vi "Jasco_UVvis.vi"() -> ()   [LabVIEW 2018]
uses:
  <vilib>/Instr/_visa.llb/VISA Configure Serial Port (Instr).vi
panel:
  in  "?":T1(tab)
  out "?":ext(graph)
  in  "SW read":bool
  out "Absorbance (ABU)":dbl
  in  "Sample rate (ms)":dbl=500.0
  in  "Wavelength (nm)":i32=350
  in  "Single wavelength absorbtion file path":path
  out "?":T2(graph)
  in  "Measure background spectra":bool
  in  "read spectrum":bool
  in  "Single wavelength absorbtion file path 2":path
  in  "stop 3":bool
  in  "stop 2":bool
  in  "flow control (0:none)":u16(ring)=1 items=["None", "XON/XOFF", "RTS/CTS", "XON/XOFF & RTS/CTS", "DTR/DSR", "XON/XOFF & DTR/DSR"]
  in  "stop bits (10: 1 bit)":u16(ring)=20 items=["1.0"=10, "1.5"=15, "2.0"=20]
  in  "parity (0:none)":enum16{"None", "Odd", "Even", "Mark", "Space"}(ring)
  in  "data bits (8)":u16=8 min=5 max=8 step=1
  in  "baud rate (9600)":u32=4800
  in  "VISA resource name":refnum<visa-resource-name>="COM4"
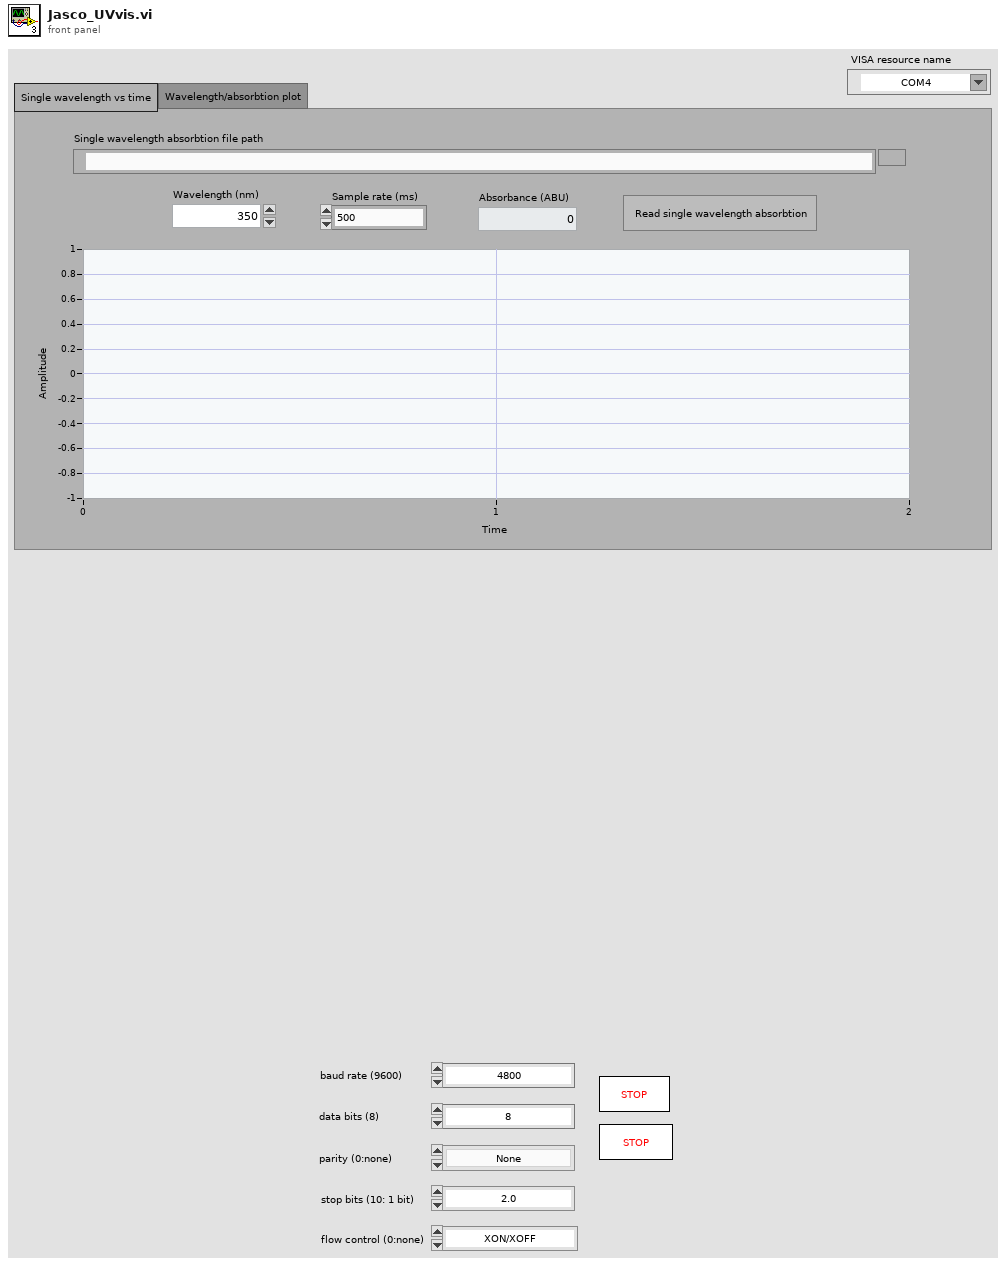
[diagram p1: front panel]
types:
  T1 = enum32{"Single wavelength vs time", "Wavelength/absorbtion plot"}
  T2 = cluster{"array type (2D Dbl)":dbl[], "array type (2D Dbl)":dbl[]}
  T3 = enum16{"open", "replace", "create", "open or create", "replace or create", "replace or create with confirmation"}
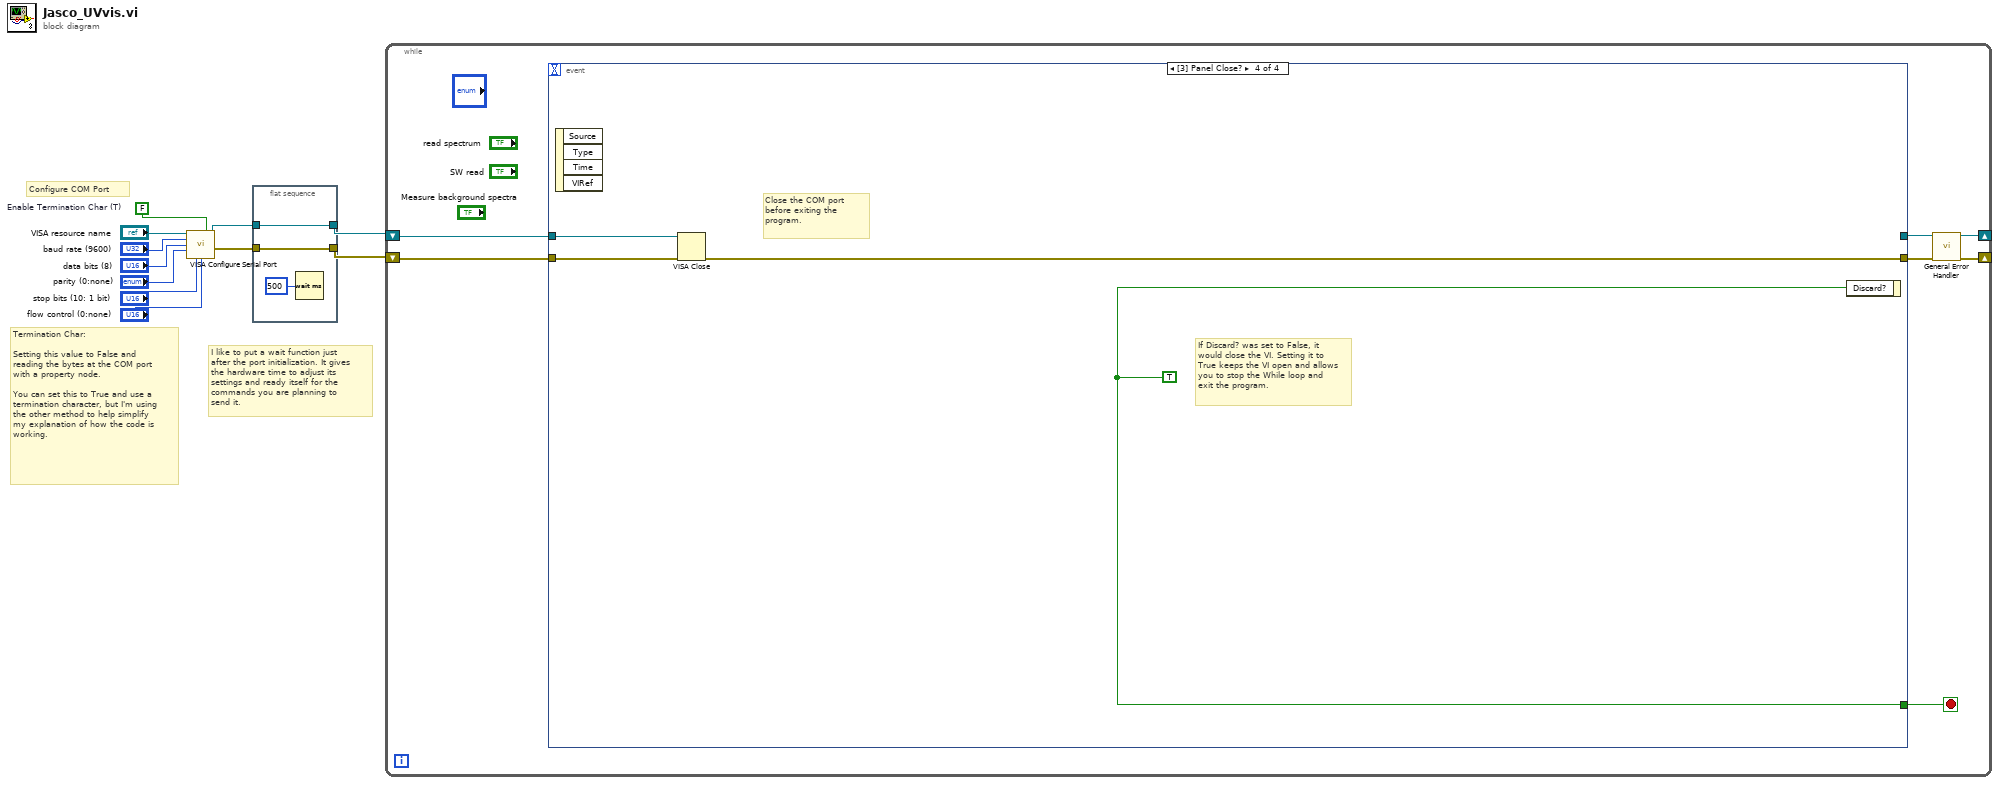
[diagram p0: block diagram]
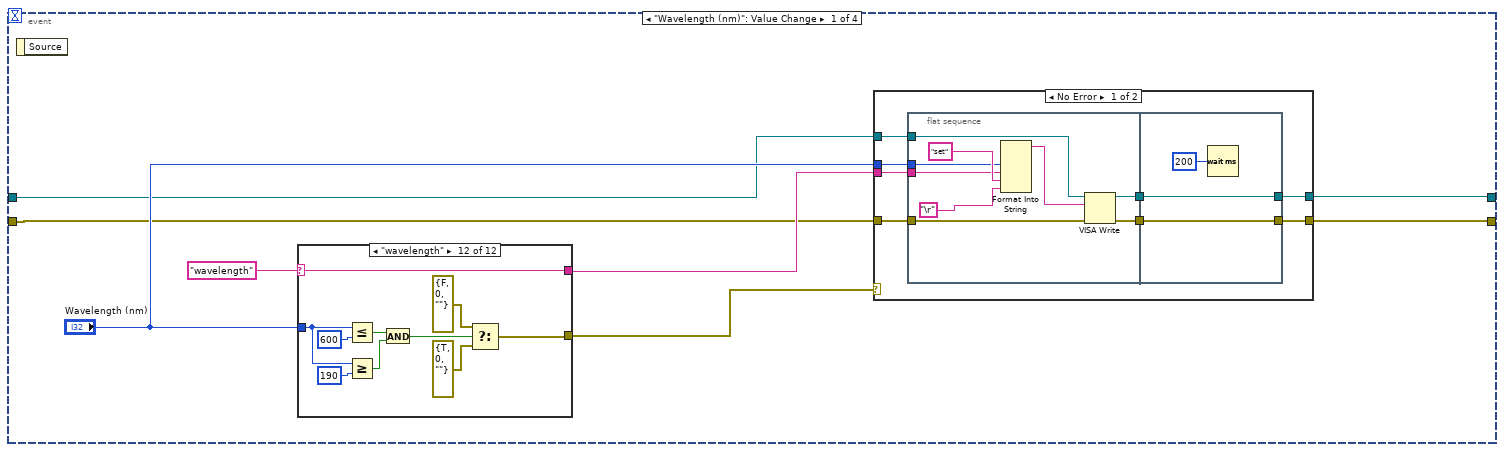
[diagram p2: hidden frame]
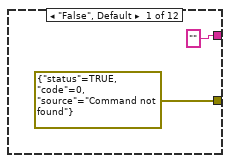
[diagram p4: hidden frame]
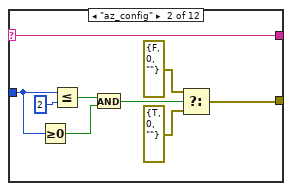
[diagram p5: hidden frame]
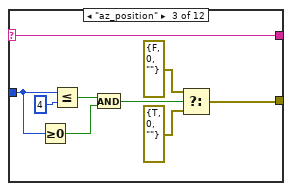
[diagram p6: hidden frame]
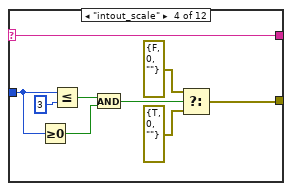
[diagram p7: hidden frame]
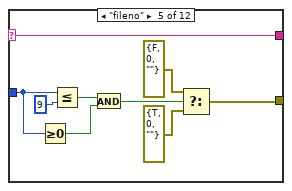
[diagram p8: hidden frame]
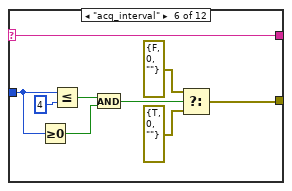
[diagram p9: hidden frame]
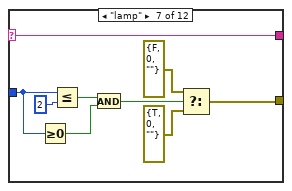
[diagram p10: hidden frame]
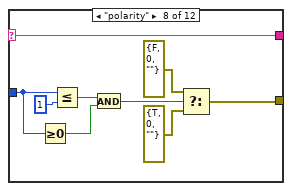
[diagram p11: hidden frame]
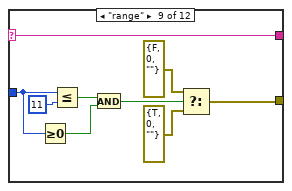
[diagram p12: hidden frame]
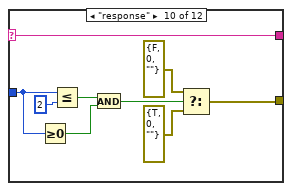
[diagram p13: hidden frame]
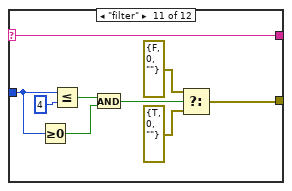
[diagram p14: hidden frame]
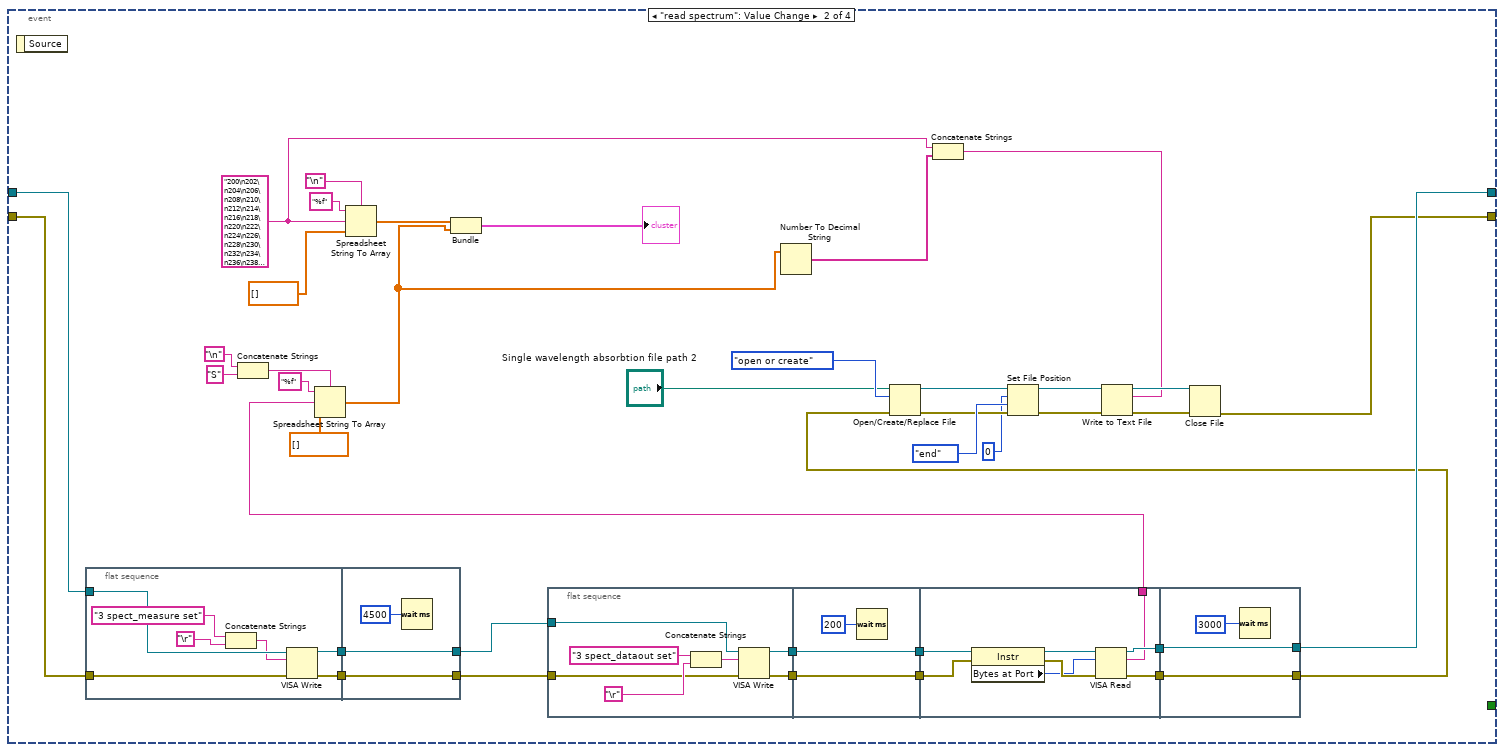
[diagram p15: hidden frame]
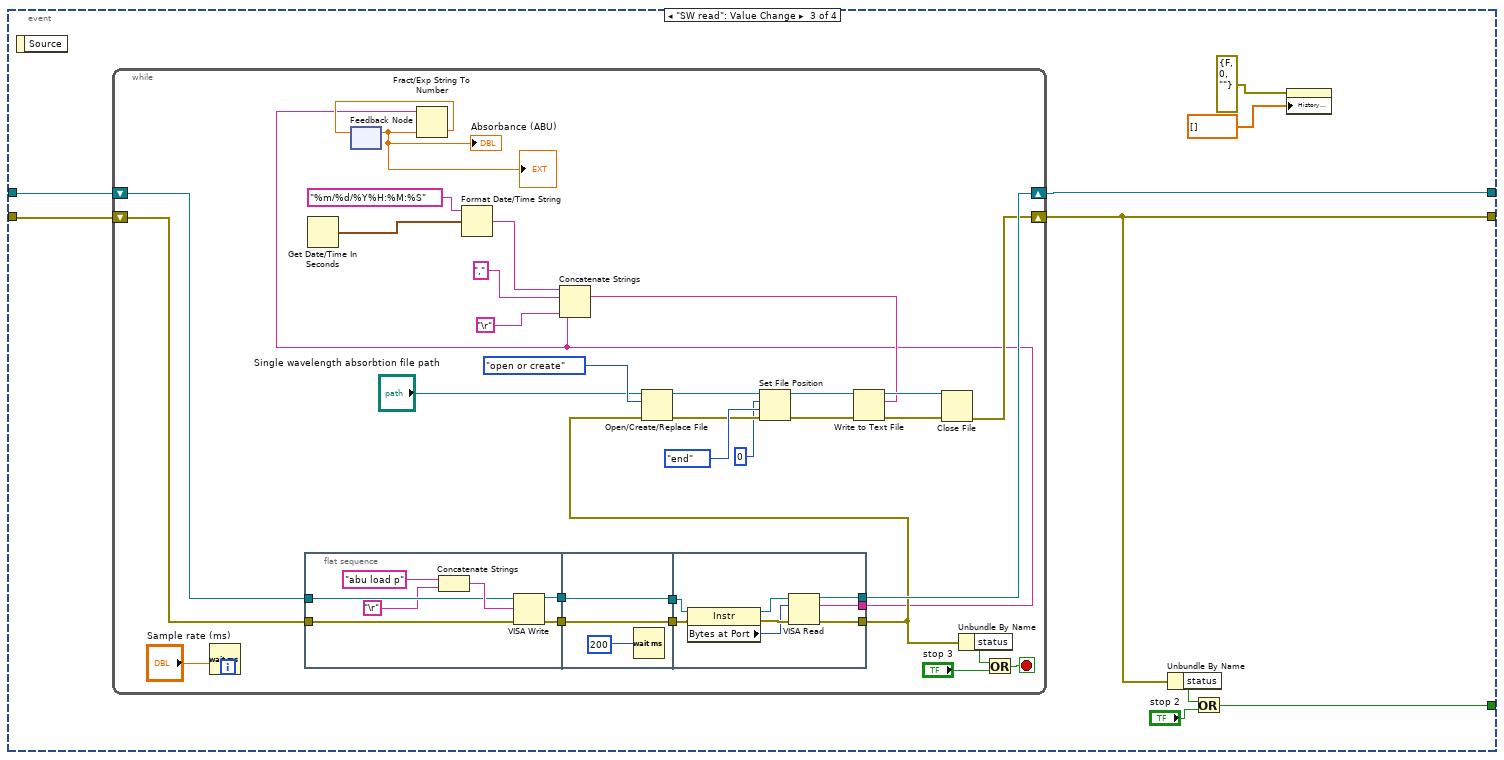
[diagram p16: hidden frame]
diagram:
  w5 = FALSE  # Enable Termination Char (T)
  # "Termination Char:\n\nSetting this value to False and reading the bytes at the COM port with a property node.\n\nYou can set this to True and use a termination character, but I'm using the other method to help simplify my explanation of how the code is working."
  # "I like to put a wait function just after the port initialization. It gives the hardware time to adjust its settings and ready itself for the commands you are planning to send it."
  # "Configure COM Port"
  n1 = call-poly "VISA Configure Serial Port"("VISA resource name"="VISA resource name", "Enable Termination\nChar (T)"=w5, "baud rate (9600)"="baud rate (9600)", "data bits (8)"="data bits (8)", "parity (0:none)"="parity (0:none)", "stop bits (10: 1 bit)"="stop bits (10: 1 bit)", "flow control (0:none)"="flow control (0:none)") -> ("VISA resource name out"=w3:refnum<visa-resource-name>, "error out"=w4:errorcluster)  [unwired: 7 in]
  n2 = flat-sequence {
    tunnel: [w13] -> w1
    tunnel: w4 -> [w13]
    tunnel: [w12] -> w2
    tunnel: w3 -> [w12]
    frame #0 {
      n3 = Wait (ms)(milliseconds to wait=u32 500) -> ()  [unwired: 1 out]
    }
  }
  n4 = while {
    shift-right: [w18] -> _
    shift-left: w2 -> [w20]
    shift-right: [w16] -> _
    shift-left: w1 -> [w19]
    stop <- w15 stop-if-true
    n5 = event shown="[3] Panel Close?" {
      selector: _ -> [_ _ _ _]
      dyn-events: _ -> [_ _ _ _]
      timeout: _ -> [_ _ _ _]
      tunnel: w20 -> [w24 w186 w231 w286]
      tunnel: w19 -> [w23 w184 w230 w285]
      tunnel: [w22 w157 w226 w284] -> w17
      tunnel: [w21 w182 w232 _] -> w18
      tunnel: [_ _ w227 w283] -> w15
      event "Wavelength (nm)": Value Change {
        n6 = event-data() -> ()  [unwired: 1 in, 1 out]
        n7 = case shown="\"wavelength\"" "wavelength" {
          selector: "wavelength" -> [_ w61 w70 w79 w88 w97 w106 w115 w124 w133 w142 w152]
          tunnel: ["" w61 w70 w79 w88 w97 w106 w115 w124 w133 w142 w152] -> w27
          tunnel: "Wavelength (nm)" -> [_ w60 w69 w78 w87 w96 w105 w114 w123 w132 w141 w144]
          tunnel: [errorcluster {"status"=TRUE, "code"=0, "source"="Command not found"} ("error in (no error)") w53 w62 w71 w80 w89 w98 w107 w116 w125 w134 w145] -> w28
          frame "False", Default {
          }
          frame "az_config" {
            n8 = Greater Or Equal To 0?(x=w60) -> (x >= 0?=w57:bool)
            n9 = Less Or Equal?(x=w60, y=2) -> (x <= y?=w58:bool)
            n10 = And(x=w58, y=w57) -> (x .and. y?=w56:bool)
            n11 = Select(t=errorcluster {"status"=FALSE, "code"=0, "source"=""} ("error in (no error)"), s=w56, f=errorcluster {"status"=TRUE, "code"=0, "source"=""} ("error in (no error)")) -> (s? t:f=w53:errorcluster)
          }
          frame "az_position" {
            n12 = Greater Or Equal To 0?(x=w69) -> (x >= 0?=w66:bool)
            n13 = Less Or Equal?(x=w69, y=4) -> (x <= y?=w67:bool)
            n14 = And(x=w67, y=w66) -> (x .and. y?=w65:bool)
            n15 = Select(t=errorcluster {"status"=FALSE, "code"=0, "source"=""} ("error in (no error)"), s=w65, f=errorcluster {"status"=TRUE, "code"=0, "source"=""} ("error in (no error)")) -> (s? t:f=w62:errorcluster)
          }
          frame "intout_scale" {
            n16 = Greater Or Equal To 0?(x=w78) -> (x >= 0?=w75:bool)
            n17 = Less Or Equal?(x=w78, y=3) -> (x <= y?=w76:bool)
            n18 = And(x=w76, y=w75) -> (x .and. y?=w74:bool)
            n19 = Select(t=errorcluster {"status"=FALSE, "code"=0, "source"=""} ("error in (no error)"), s=w74, f=errorcluster {"status"=TRUE, "code"=0, "source"=""} ("error in (no error)")) -> (s? t:f=w71:errorcluster)
          }
          frame "fileno" {
            n20 = Greater Or Equal To 0?(x=w87) -> (x >= 0?=w84:bool)
            n21 = Less Or Equal?(x=w87, y=9) -> (x <= y?=w85:bool)
            n22 = And(x=w85, y=w84) -> (x .and. y?=w83:bool)
            n23 = Select(t=errorcluster {"status"=FALSE, "code"=0, "source"=""} ("error in (no error)"), s=w83, f=errorcluster {"status"=TRUE, "code"=0, "source"=""} ("error in (no error)")) -> (s? t:f=w80:errorcluster)
          }
          frame "acq_interval" {
            n24 = Greater Or Equal To 0?(x=w96) -> (x >= 0?=w93:bool)
            n25 = Less Or Equal?(x=w96, y=4) -> (x <= y?=w94:bool)
            n26 = And(x=w94, y=w93) -> (x .and. y?=w92:bool)
            n27 = Select(t=errorcluster {"status"=FALSE, "code"=0, "source"=""} ("error in (no error)"), s=w92, f=errorcluster {"status"=TRUE, "code"=0, "source"=""} ("error in (no error)")) -> (s? t:f=w89:errorcluster)
          }
          frame "lamp" {
            n28 = Greater Or Equal To 0?(x=w105) -> (x >= 0?=w102:bool)
            n29 = Less Or Equal?(x=w105, y=2) -> (x <= y?=w103:bool)
            n30 = And(x=w103, y=w102) -> (x .and. y?=w101:bool)
            n31 = Select(t=errorcluster {"status"=FALSE, "code"=0, "source"=""} ("error in (no error)"), s=w101, f=errorcluster {"status"=TRUE, "code"=0, "source"=""} ("error in (no error)")) -> (s? t:f=w98:errorcluster)
          }
          frame "polarity" {
            n32 = Greater Or Equal To 0?(x=w114) -> (x >= 0?=w111:bool)
            n33 = Less Or Equal?(x=w114, y=1) -> (x <= y?=w112:bool)
            n34 = And(x=w112, y=w111) -> (x .and. y?=w110:bool)
            n35 = Select(t=errorcluster {"status"=FALSE, "code"=0, "source"=""} ("error in (no error)"), s=w110, f=errorcluster {"status"=TRUE, "code"=0, "source"=""} ("error in (no error)")) -> (s? t:f=w107:errorcluster)
          }
          frame "range" {
            n36 = Greater Or Equal To 0?(x=w123) -> (x >= 0?=w120:bool)
            n37 = Less Or Equal?(x=w123, y=11) -> (x <= y?=w121:bool)
            n38 = And(x=w121, y=w120) -> (x .and. y?=w119:bool)
            n39 = Select(t=errorcluster {"status"=FALSE, "code"=0, "source"=""} ("error in (no error)"), s=w119, f=errorcluster {"status"=TRUE, "code"=0, "source"=""} ("error in (no error)")) -> (s? t:f=w116:errorcluster)
          }
          frame "response" {
            n40 = Greater Or Equal To 0?(x=w132) -> (x >= 0?=w129:bool)
            n41 = Less Or Equal?(x=w132, y=2) -> (x <= y?=w130:bool)
            n42 = And(x=w130, y=w129) -> (x .and. y?=w128:bool)
            n43 = Select(t=errorcluster {"status"=FALSE, "code"=0, "source"=""} ("error in (no error)"), s=w128, f=errorcluster {"status"=TRUE, "code"=0, "source"=""} ("error in (no error)")) -> (s? t:f=w125:errorcluster)
          }
          frame "filter" {
            n44 = Greater Or Equal To 0?(x=w141) -> (x >= 0?=w138:bool)
            n45 = Less Or Equal?(x=w141, y=4) -> (x <= y?=w139:bool)
            n46 = And(x=w139, y=w138) -> (x .and. y?=w137:bool)
            n47 = Select(t=errorcluster {"status"=FALSE, "code"=0, "source"=""} ("error in (no error)"), s=w137, f=errorcluster {"status"=TRUE, "code"=0, "source"=""} ("error in (no error)")) -> (s? t:f=w134:errorcluster)
          }
          frame "wavelength" {
            n48 = Less Or Equal?(x=w144, y=600) -> (x <= y?=w150:bool)
            n49 = Greater Or Equal?(x=w144, y=190) -> (x >= y?=w149:bool)
            n50 = And(x=w150, y=w149) -> (x .and. y?=w148:bool)
            n51 = Select(t=errorcluster {"status"=FALSE, "code"=0, "source"=""} ("error in (no error)"), s=w148, f=errorcluster {"status"=TRUE, "code"=0, "source"=""} ("error in (no error)")) -> (s? t:f=w145:errorcluster)
          }
        }
        n52 = case shown="No Error" w28 {
          tunnel: w24 -> [w34 w49]
          tunnel: [w33 w49] -> w21
          tunnel: [w32 w50] -> w22
          tunnel: w23 -> [w31 w50]
          tunnel: w27 -> [w30 _]
          tunnel: "Wavelength (nm)" -> [w29 _]
          frame No Error {
            n53 = flat-sequence {
              tunnel: w30 -> [w39]
              tunnel: w31 -> [w45]
              tunnel: w34 -> [w44]
              tunnel: [w43] -> w36
              tunnel: [w42] -> w35
              tunnel: w29 -> [w38]
              tunnel: [w47] -> w32
              tunnel: w36 -> [w47]
              tunnel: [w46] -> w33
              tunnel: w35 -> [w46]
              frame #0 {
                n54 = Format Into String(w38, w39, "set" ("string"), "\r") -> (resulting string=w40:string)  [unwired: 3 in, 1 out]
                n55 = VISA Write(VISA resource name=w44, write buffer=w40, error in (no error)=w45) -> (VISA resource name out=w42:refnum<visa-resource-name>, error out=w43:errorcluster)  [unwired: 1 out]
              }
              frame #1 {
                n56 = Wait (ms)(milliseconds to wait=u32 200) -> ()  [unwired: 1 out]
              }
            }
          }
          frame Error {
          }
        }
      }
      event "read spectrum": Value Change {
        w156 = "200\n202\n204\n206\n208\n210\n212\n214\n216\n218\n220\n222\n224\n226\n228\n230\n232\n234\n236\n238\n240\n242\n244\n246\n248\n250\n252\n254\n256\n258\n260\n262\n264\n266\n268\n270\n272\n274\n276\n278\n280\n282\n284\n286\n288\n290\n292\n294\n296\n298\n300\n302\n304\n306\n308\n310\n312\n314\n316\n318\n320\n322\n324\n326\n328\n330\n332\n334\n336\n338\n340\n342\n344\n346\n348\n350\n352\n354\n356\n358\n360\n362\n364\n366\n368\n370\n372\n374\n376\n378\n380\n382\n384\n386\n388\n390\n392\n394\n396\n398\n400\n402\n404\n406\n408\n410\n412\n414\n416\n418\n420\n422\n424\n426\n428\n430\n432\n434\n436\n438\n440\n442\n444\n446\n448\n450\n452\n454\n456\n458\n460\n462\n464\n466\n468\n470\n472\n474\n476\n478\n480\n482\n484\n486\n488\n490\n492\n494\n496\n498\n500\n502\n504\n506\n508\n510\n512\n514\n516\n518\n520\n522\n524\n526\n528\n530\n532\n534\n536\n538\n540\n542\n544\n546\n548\n550\n552\n554\n556\n558\n560\n562\n564\n566\n568\n570\n572\n574\n576\n578\n580\n582\n584\n586\n588\n590\n592\n594\n596\n598\n600\n602\n"
        n57 = event-data() -> ()  [unwired: 1 in, 1 out]
        n58 = flat-sequence {
          tunnel: w184 -> [w199]
          tunnel: w186 -> [w198]
          tunnel: [w197] -> w188
          tunnel: [w196] -> w187
          tunnel: [w201] -> w183
          tunnel: w188 -> [w201]
          tunnel: [w200] -> w185
          tunnel: w187 -> [w200]
          frame #0 {
            n59 = Concatenate Strings("3 spect_measure set" ("string"), "\r") -> (w194:string)
            n60 = VISA Write(VISA resource name=w198, write buffer=w194, error in (no error)=w199) -> (VISA resource name out=w196:refnum<visa-resource-name>, error out=w197:errorcluster)  [unwired: 1 out]
          }
          frame #1 {
            n61 = Wait (ms)(milliseconds to wait=u32 4500) -> ()  [unwired: 1 out]
          }
        }
        n62 = Concatenate Strings("\n", "S") -> (w176:string)
        n63 = Spreadsheet String To Array(delimiter (Tab)=w176, format string="%f", spreadsheet string=w169, array type (2D Dbl)=dbl[] []) -> (array=w155:dbl[])
        n64 = Spreadsheet String To Array(delimiter (Tab)="\n", format string="%f", spreadsheet string=w156, array type (2D Dbl)=dbl[] []) -> (array=w170:dbl[])
        n65 = Bundle("array type (2D Dbl)"=w170, "array type (2D Dbl)"=w155) -> (→"?":T2)  [unwired: 1 in]
        n66 = flat-sequence {
          tunnel: [w207] -> w192
          tunnel: [w206] -> w191
          tunnel: w183 -> [w203]
          tunnel: w185 -> [w208]
          tunnel: w192 -> [w211]
          tunnel: w191 -> [w210]
          tunnel: [w211] -> w190
          tunnel: [w210] -> w189
          tunnel: w190 -> [w220]
          tunnel: w189 -> [w218]
          tunnel: [w216] -> w181
          tunnel: [w214] -> w180
          tunnel: [w213] -> w169
          tunnel: [w222] -> w158
          tunnel: [w223] -> w182
          tunnel: w181 -> [w223]
          tunnel: w180 -> [w222]
          frame #0 {
            n67 = Concatenate Strings("3 spect_dataout set" ("string"), "\r") -> (w209:string)
            n68 = VISA Write(VISA resource name=w208, write buffer=w209, error in (no error)=w203) -> (VISA resource name out=w206:refnum<visa-resource-name>, error out=w207:errorcluster)  [unwired: 1 out]
          }
          frame #1 {
            n69 = Wait (ms)(milliseconds to wait=u32 200) -> ()  [unwired: 1 out]
          }
          frame #2 {
            n70 = property class="Instr"(reference=w218, error in=w220) -> (reference out=w217:refnum<visa-resource-name>, error out=w219:errorcluster, "Bytes at Port"=w215:u32)
            n71 = VISA Read(VISA resource name=w217, byte count=w215, error in (no error)=w219) -> (VISA resource name out=w216:refnum<visa-resource-name>, read buffer=w213:string, error out=w214:errorcluster)  [unwired: 1 out]
          }
          frame #3 {
            n72 = Wait (ms)(milliseconds to wait=u32 3000) -> ()  [unwired: 1 out]
          }
        }
        n73 = Number To Decimal String(number=w155) -> (decimal integer string=w154:string[])  [unwired: 1 in]
        n74 = Open/Create/Replace File(file path (use dialog)="Single wavelength absorbtion file path 2", error in=w158, operation (0:open)=T3."open or create") -> (refnum out=w162:refnum<file>, error out=w161:errorcluster)  [unwired: 3 in, 1 out]
        n75 = Concatenate Strings(w156, w154) -> (w153:string)
        n76 = Set File Position(offset (in bytes) (0)=i64 0, refnum=w162, from (0:start)=enum16{"start", "end", "current"}."end", error in=w161) -> (refnum out=w166:refnum<file>, error out=w167:errorcluster)
        n77 = Write to Text File(file (use dialog)=w166, text=w153, error in=w167) -> (refnum out=w164:refnum<file>, error out=w165:errorcluster)  [unwired: 1 in, 1 out]
        n78 = Close File(refnum=w164, error in=w165) -> (error out=w157:errorcluster)  [unwired: 1 out]
      }
      event "SW read": Value Change {
        n79 = event-data() -> ()  [unwired: 1 in, 1 out]
        n80 = while {
          shift-right: [w260] -> w232
          shift-left: w231 -> [w233]
          shift-right: [w241] -> w226
          shift-left: w230 -> [w238]
          stop <- w257 stop-if-true
          n81 = Wait (ms)(milliseconds to wait="Sample rate (ms)") -> ()  [unwired: 1 out]
          n82 = flat-sequence {
            tunnel: w238 -> [w265]
            tunnel: w233 -> [w270]
            tunnel: [w269] -> w264
            tunnel: [w268] -> w263
            tunnel: w264 -> [w273]
            tunnel: w263 -> [w272]
            tunnel: [w273] -> w262
            tunnel: [w272] -> w261
            tunnel: w262 -> [w281]
            tunnel: w261 -> [w279]
            tunnel: [w282] -> w242
            tunnel: [w277] -> w260
            tunnel: [w275] -> w236
            frame #0 {
              n83 = Concatenate Strings("abu load p" ("string"), "\r") -> (w271:string)
              n84 = VISA Write(VISA resource name=w270, write buffer=w271, error in (no error)=w265) -> (VISA resource name out=w268:refnum<visa-resource-name>, error out=w269:errorcluster)  [unwired: 1 out]
            }
            frame #1 {
              n85 = Wait (ms)(milliseconds to wait=u32 200) -> ()  [unwired: 1 out]
            }
            frame #2 {
              n86 = property class="Instr"(reference=w279, error in=w281) -> (reference out=w278:refnum<visa-resource-name>, error out=w280:errorcluster, "Bytes at Port"=w276:u32)
              n87 = VISA Read(VISA resource name=w278, byte count=w276, error in (no error)=w280) -> (VISA resource name out=w277:refnum<visa-resource-name>, read buffer=w275:string, error out=w282:errorcluster)  [unwired: 1 out]
            }
          }
          n88 = Get Date/Time In Seconds() -> (seconds since 1Jan1904=w255:timestamp)
          n89 = feedback #1() -> (w235:ext)  [unwired: 1 in]
          "Absorbance (ABU)" <- w235
          "?" <- w235
          n90 = Fract/Exp String To Number(string=w236, default (0 dbl)=w235) -> (number=w239:ext)  [unwired: 2 in, 1 out]
          n91 = feedback-in #1(w239) -> ()
          n92 = Format Date/Time String(time format string (%c)="%m/%d/%Y%H:%M:%S", seconds (now)=w255) -> (date/time string=w253:string)  [unwired: 1 in]
          n93 = Concatenate Strings(w253, ",", w236, "\r") -> (w240:string)
          n94 = Open/Create/Replace File(file path (use dialog)="Single wavelength absorbtion file path", error in=w242, operation (0:open)=T3."open or create") -> (refnum out=w245:refnum<file>, error out=w244:errorcluster)  [unwired: 3 in, 1 out]
          n95 = Set File Position(offset (in bytes) (0)=i64 0, refnum=w245, from (0:start)=enum16{"start", "end", "current"}."end", error in=w244) -> (refnum out=w249:refnum<file>, error out=w250:errorcluster)
          n96 = Write to Text File(file (use dialog)=w249, text=w240, error in=w250) -> (refnum out=w247:refnum<file>, error out=w248:errorcluster)  [unwired: 1 in, 1 out]
          n97 = Close File(refnum=w247, error in=w248) -> (error out=w241:errorcluster)  [unwired: 1 out]
          n98 = Unbundle By Name(w242) -> ("status"=w258:bool)
          n99 = Or(x=w258, y="stop 3") -> (x .or. y?=w257:bool)
        }
        n100 = Unbundle By Name(w226) -> ("status"=w229:bool)
        n101 = Or(x=w229, y="stop 2") -> (x .or. y?=w227:bool)
        n102 = property class="WFChart (strict)"(error in=errorcluster {"status"=FALSE, "code"=0, "source"=""} ("error in (no error)"), "History Data"=ext[] []) -> ()  [unwired: 1 in, 2 out]
      }
      event Panel Close? {
        w283 = TRUE ("Discard?")
        # "If Discard? was set to False, it would close the VI. Setting it to True keeps the VI open and allows you to stop the While loop and exit the program."
        # "Close the COM port before exiting the program."
        n103 = event-data() -> ()  [unwired: 1 in, 4 out]
        n104 = VISA Close(VISA resource name=w286, error in (no error)=w285) -> (error out=w284:errorcluster)
        n105 = event-data("Discard?"=w283) -> ()  [unwired: 1 in, 1 out]
      }
    }
    n106 = call <vilib>:"General Error Handler.vi"("error in (no error)"=w17) -> ("error out"=w16:errorcluster)  [unwired: 10 in, 4 out]
  }
